vi "Init.vi"(8 "error in (no error)":errorcluster, 11 "TCP Text Writer in":refnum<class "TCP Text Writer.lvclass">) -> (0 "error out":errorcluster, 3 "TCP Text Writer out":refnum<class "TCP Text Writer.lvclass">)   [LabVIEW 2026, in "TALOS.lvlib" / "TCP Text Writer.lvlib" / "TCP Text Writer.lvclass"]
uses:
  TCP Text Writer.lvclass
  C:/LabVIEW Code/TALOS/talos/Father of all uServices/Father of all uServices/Father of all uServices.lvclass
  Father of all uServices/Father of all uServices/Father of all uServices.lvclass/Father of all uServices.ctl
  Ancestor/Ancestor/Ancestor.lvclass/Ancestor.ctl
  Support VIs/Substitute Error.vi
  Support VIs/Generate Error.vi
  FGV/Error Memory/Get Error Description.vi
  Support VIs/Get PC name.vi
  Ancestor/Ancestor/Read ID.vi
  Support VIs/Get Class Name.vi
  <vilib>/Utility/error.llb/Clear Errors.vi
  FGV/Error Memory/Error Memory Core.vi
  <vilib>/AdvancedString/Delimited String to 1D String Array.vi
  <vilib>/AdvancedString/Delimited String to 1D String Array (string).vi
  Support VIs/Circus Root Path.vi
  FGV/Error Memory/Error Crt Lvl checker.vi
  FGV/Error Memory/Error Memory Core.vi/40c8088d-b597-4017-91af-faa98e00292e.vi
  FGV/Error Memory/Error Memory Core.vi/d4a3ab98-063c-4e44-b43d-fbdcfe6c2be2.vi
  Support VIs/Global Memory.vi
  <vilib>/Utility/LVClass/Get LV Class Name.vi
  Support VIs/Is in Packed Library.vi
  Support VIs/TALOS Root path.vi
  Support VIs/Read CSV worksheet.vi
  Support VIs/Global Constants.vi
  <vilib>/Utility/error.llb/General Error Handler.vi
  Support VIs/Error Log.vi
  TCP Writer/TCP Writer/TCP Writer.lvclass
  Ancestor/Ancestor/Ancestor.lvclass
  <vilib>/Comparison/Equal/Equal Functor/Equal Functor.lvclass
  Father of all uServices/Father of all uServices/Father of all uServices.lvclass
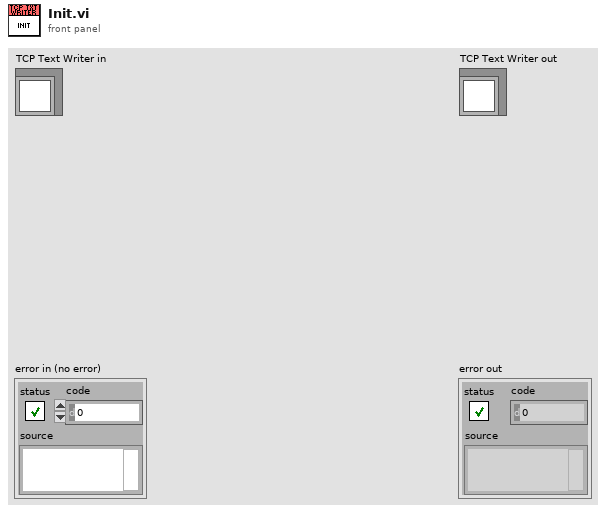
[diagram p1: front panel]
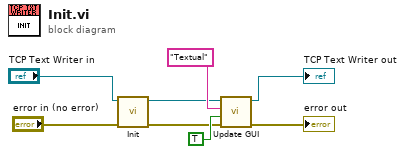
[diagram p0: block diagram]
diagram:
  n1 = call-parent "Init.vi"("error in (no error)"="error in (no error)", "TCP Writer in"="TCP Text Writer in") -> ("error out"=w3:errorcluster, "TCP Writer out"=w4:refnum<class "TCP Text Writer.lvclass">)  [unwired: 8 in]
  n2 = call "Update GUI.vi"("error in (no error)"=w3, "Data"=TRUE ("Textual"), "GUI Item Name"="Textual", "uService Template in"=w4) -> ("error out"=→"error out":errorcluster, "uService Template out"=→"TCP Text Writer out":refnum<class "TCP Text Writer.lvclass">)  [unwired: 6 in]
